vi "Prog12.vi"() -> ()   [LabVIEW 2021]
panel:
  out "Array 4":string[](array[string])
  out "Array 3":i32[](array[numeric])
  out "Array 2":string[](array[string])
  out "Array":i32[](array[numeric])
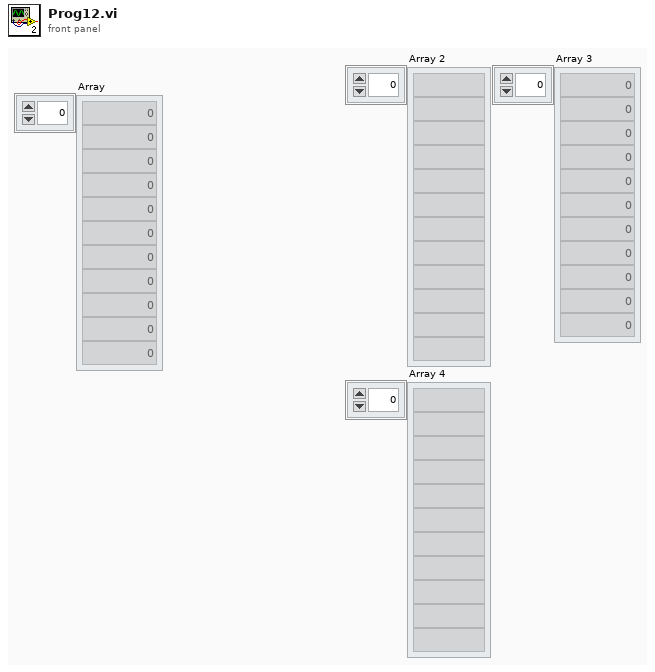
[diagram p1: front panel]
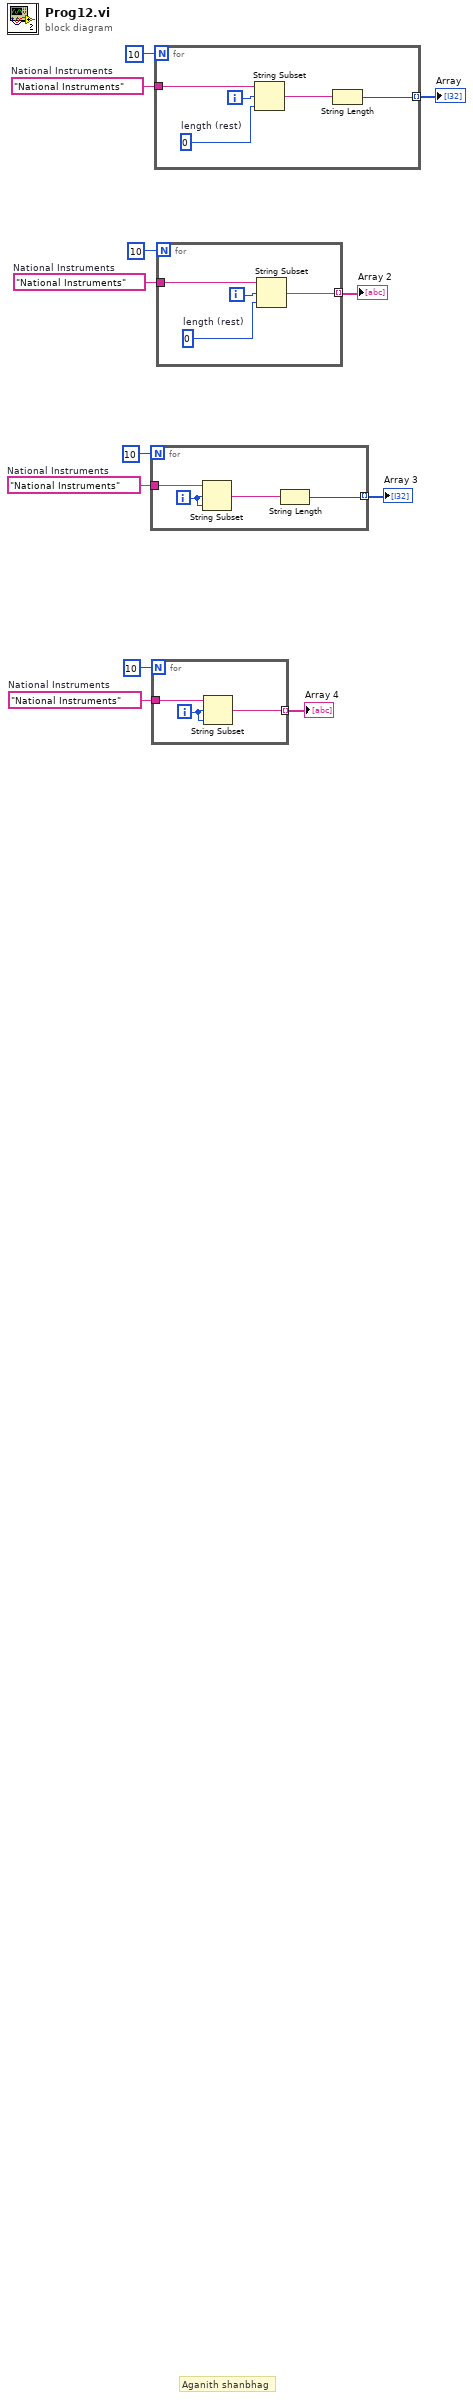
[diagram p0: block diagram]
diagram:
  w3 = "National Instruments"  # National Instruments
  w6 = "National Instruments"  # National Instruments
  w9 = "National Instruments"  # National Instruments
  w12 = "National Instruments"  # National Instruments
  # "Aganith shanbhag"
  n1 = for {
    N: 10 -> [_]
    tunnel: w6 -> [w16]
    tunnel: [w14] -> w5 mode=indexing
    i -> [w13]
    n2 = String Subset(string=w16, offset (0)=w13, length (rest)=w13) -> (substring=w15:string)
    n3 = String Length(string=w15) -> (length=w14:i32)
  }
  "Array 3" <- w5
  n4 = for {
    N: 10 -> [_]
    tunnel: w3 -> [w19]
    tunnel: [w17] -> w1 mode=indexing
    i -> [w18]
    n5 = String Subset(string=w19, offset (0)=w18, length (rest)=w18) -> (substring=w17:string)
  }
  "Array 4" <- w1
  n6 = for {
    N: 10 -> [_]
    tunnel: w12 -> [w24]
    tunnel: [w20] -> w11 mode=indexing
    i -> [w23]
    w22 = 0  # length (rest)
    n7 = String Subset(string=w24, offset (0)=w23, length (rest)=w22) -> (substring=w21:string)
    n8 = String Length(string=w21) -> (length=w20:i32)
  }
  "Array" <- w11
  n9 = for {
    N: 10 -> [_]
    tunnel: w9 -> [w28]
    tunnel: [w25] -> w7 mode=indexing
    i -> [w27]
    w26 = 0  # length (rest)
    n10 = String Subset(string=w28, offset (0)=w27, length (rest)=w26) -> (substring=w25:string)
  }
  "Array 2" <- w7
